vi "Data Analysis.COnvert JSON to CSV.vi"(8 "error in (no error)":errorcluster, 10 "Output Folder":path, 11 "Input Folder":path) -> (0 "error out":errorcluster)   [LabVIEW 2018]
uses:
  Common/Utils/Reports/Report.Result Data JSON V2.0.0.ctl
  Common/Utils/Reports/Report.Result Test Event.ctl
  Common/Utils/Reports/Report.Result State.ctl
  Common/Utils/Reports/Report.Result UUTInfo.ctl
  Common/Utils/Reports/Report.Result Test Station.ctl
  Common/Utils/Reports/Report.Result Test Sequence.ctl
  Common/Utils/Reports/Report.Result Measurement JSON Safe.ctl
  Common/Utils/Reports/Report.Result DataObject.ctl
  <vilib>/KATE/Files/File Utils.lvlib
  <vilib>/zip/NI_Unzip.lvlib
panel:
  in  "Abort":bool
  out "ZipCnt":i32
  out "JSONCnt":i32
  out "ZIP Files In":path[](array[path])
  out "Files Out":path[](array[path])
  out "JSON Files In":path[](array[path])
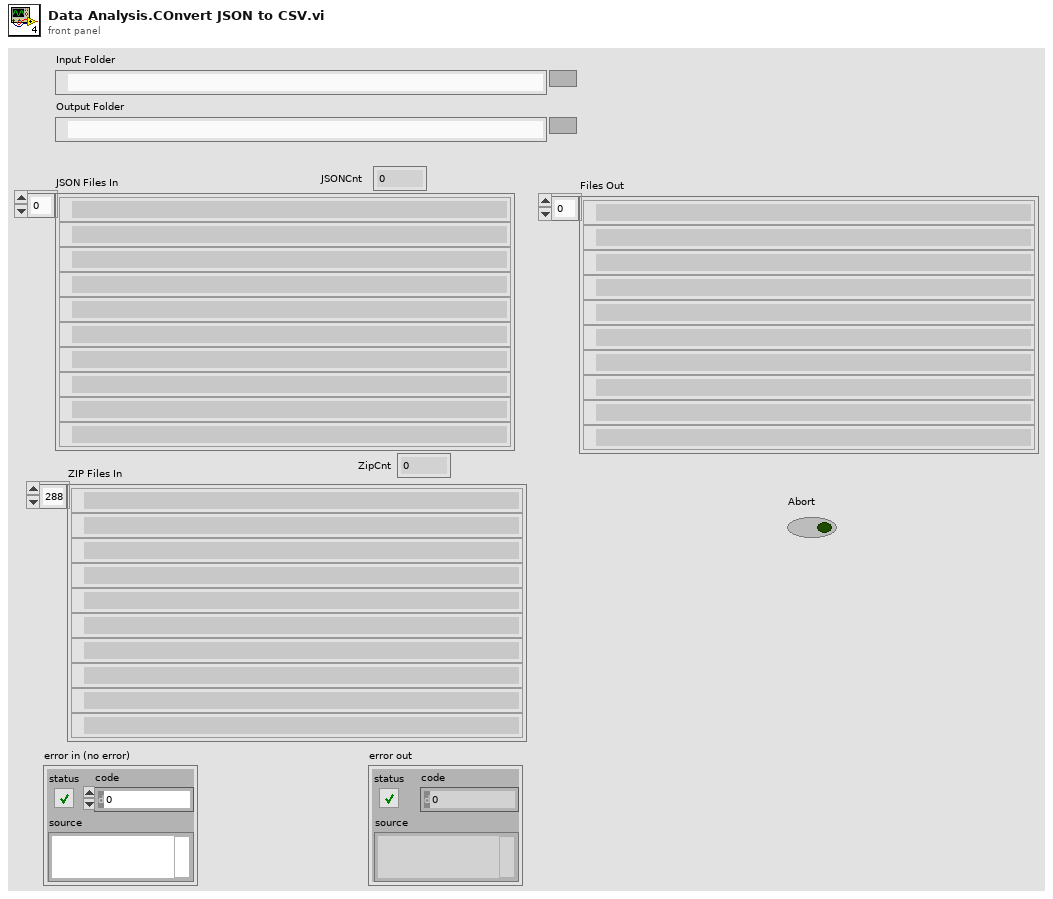
[diagram p1: front panel]
types:
  T1 = typedef "Report.Result Data JSON V2.0.0.ctl" = cluster{"Type":string, "Version":string, "TestEvent":T2, "UUTInfo":T4, "Station":T5, "TestSequence":T6, "ResultData":T7[], "DataObjs":T8[]}
  T2 = typedef "Report.Result Test Event.ctl" = cluster{"ProcessStep":string, "StartTime":string, "EndTime":string, "Mode":string, "Operator":string, "Comment":string, "Result":T3}
  T3 = typedef "Report.Result State.ctl" = cluster{"State":string, "Code":i32, "Desc":string, "Details":string}
  T4 = typedef "Report.Result UUTInfo.ctl" = cluster{"Product":string, "Description":string, "PN":string, "SN":string, "LotNumber":string, "DateCode":string, "AltID":string, "Revision":string, "Properties":cluster{"Name":string, "Value":string}[]}
  T5 = typedef "Report.Result Test Station.ctl" = cluster{"Name":string, "Location":string, "ConfigID":string, "PCName":string, "Slot":string}
  T6 = typedef "Report.Result Test Sequence.ctl" = cluster{"Name":string, "Setup":cluster{"Name":string, "Value":string}[]}
  T7 = typedef "Report.Result Measurement JSON Safe.ctl" = cluster{"Cnt":i32, "Step":string, "Category":string, "Name":string, "Value":string, "Units":string, "LimType":string, "LL":string, "UL":string, "Time":string, "Result":T3}
  T8 = typedef "Report.Result DataObject.ctl" = cluster{"Cnt":i32, "Step":string, "Category":string, "Name":string, "Type":string, "FileName":string, "Time":string}
  T9 = cluster{"JSON Files In":path[], "ZIP Files In":path[]}
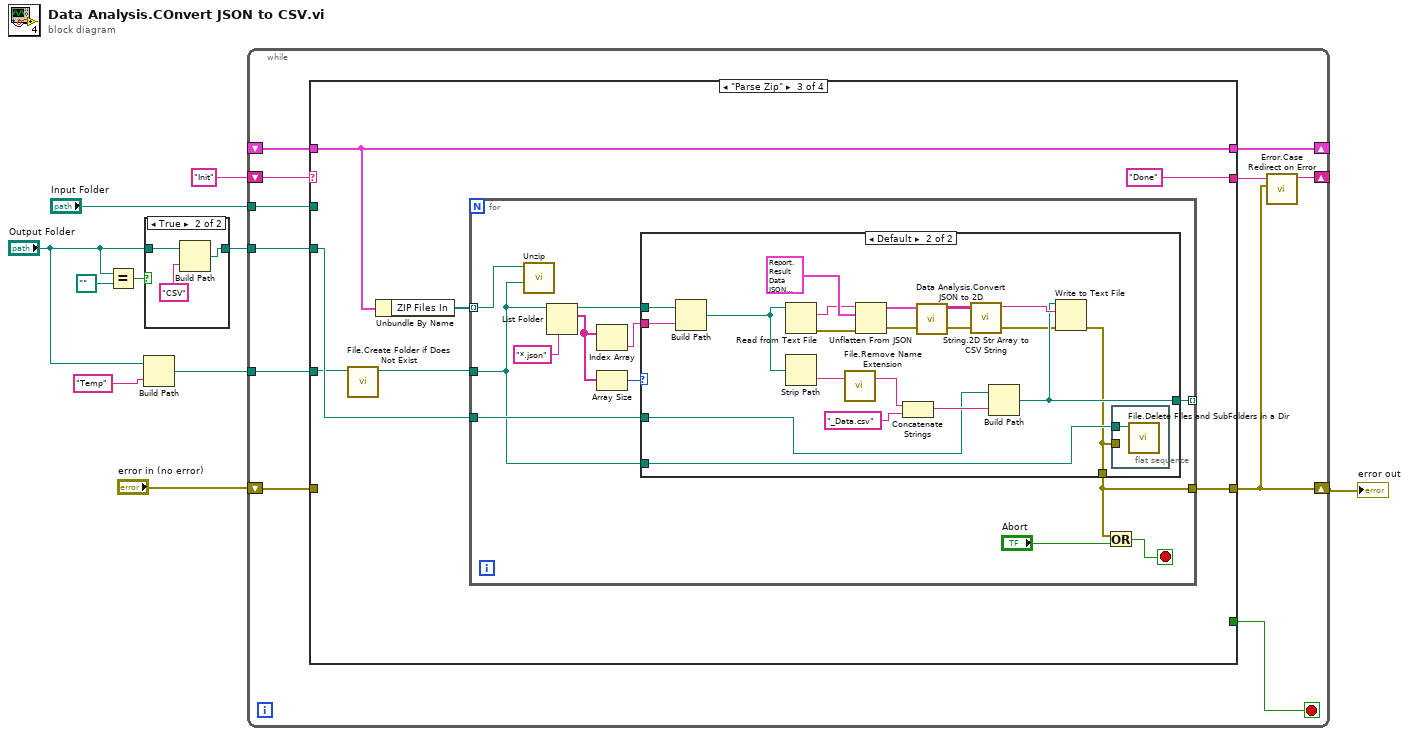
[diagram p0: block diagram]
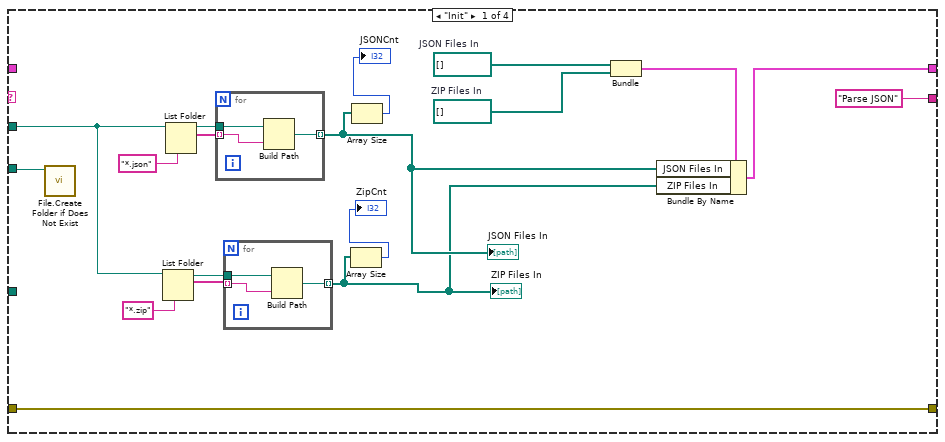
[diagram p3: hidden frame]
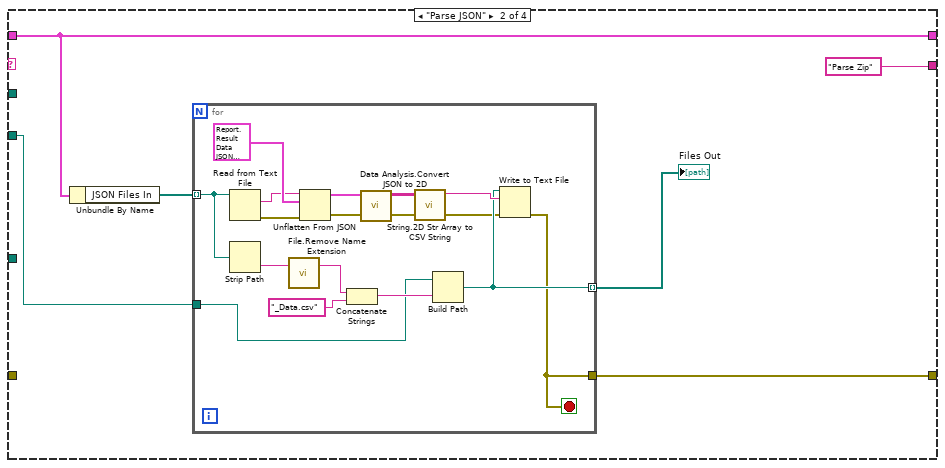
[diagram p4: hidden frame]
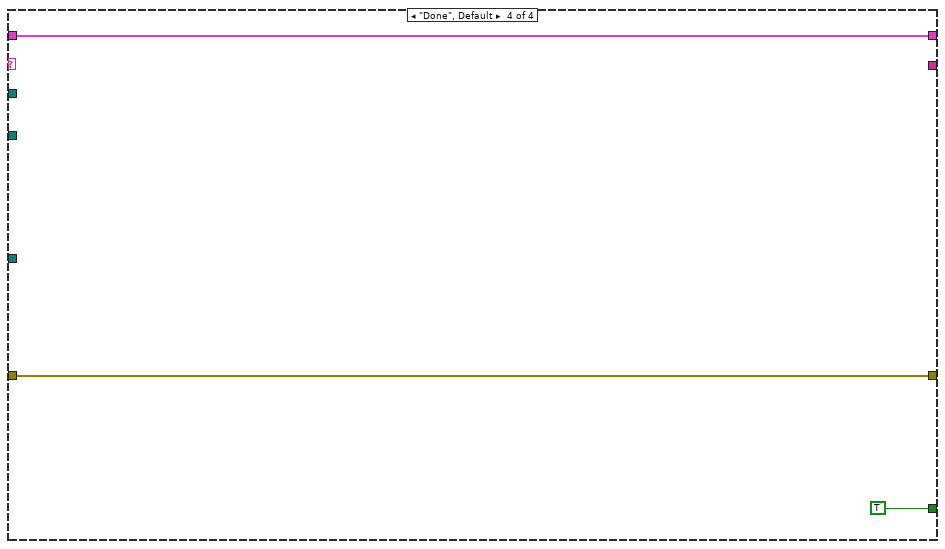
[diagram p6: hidden frame]
diagram:
  n1 = Equal?(x="Output Folder", y=path "") -> (x = y?=w6:bool)
  n2 = Build Path(base path="Output Folder", name or relative path="Temp") -> (appended path=w1:path)
  n3 = case shown="True" w6 {
    tunnel: "Output Folder" -> [w11 w13]
    tunnel: [w11 w12] -> w7
    frame False {
    }
    frame True {
      n4 = Build Path(base path=w13, name or relative path="CSV") -> (appended path=w12:path)
    }
  }
  n5 = while {
    tunnel: "Input Folder" -> [w25]
    tunnel: w7 -> [w24]
    shift-right: [w18] -> _
    shift-left: "Init" -> [w23]
    shift-right: [w21] -> _
    shift-left: _ -> [w20]
    shift-right: [w17] -> w4
    shift-left: "error in (no error)" -> [w16]
    tunnel: w1 -> [w15]
    stop <- w22 stop-if-true
    n6 = case shown="\"Parse Zip\"" w23 {
      tunnel: w25 -> [w40 _ _ _]
      tunnel: w24 -> [w43 w52 w74 _]
      tunnel: ["Parse JSON" "Parse Zip" "Done" _] -> w19
      tunnel: [_ _ _ TRUE] -> w22
      tunnel: [w30 w54 w76 w110] -> w21
      tunnel: w20 -> [_ w54 w76 w110]
      tunnel: [w32 w50 w73 w109] -> w17
      tunnel: w16 -> [w32 _ _ w109]
      tunnel: w15 -> [_ _ w72 _]
      frame "Init" {
        w33 = path[] []  # ZIP Files In
        w34 = path[] []  # JSON Files In
        n7 = call <vilib>:"File.Create Folder if Does Not Exist.vi"("Path"=w43) -> ()  [unwired: 8 in, 3 out]
        n8 = List Folder(path=w40, pattern="*.zip") -> (path out=w37:path, filenames=w36:string[])  [unwired: 2 in, 2 out]
        n9 = List Folder(path=w40, pattern="*.json") -> (path out=w39:path, filenames=w38:string[])  [unwired: 2 in, 2 out]
        n10 = for {
          tunnel: w39 -> [w49]
          tunnel: w38 -> [w48] mode=indexing
          tunnel: [w47] -> w29 mode=indexing
          n11 = Build Path(base path=w49, name or relative path=w48) -> (appended path=w47:path)
        }
        "JSON Files In" <- w29
        n12 = for {
          tunnel: w37 -> [w46]
          tunnel: w36 -> [w45] mode=indexing
          tunnel: [w44] -> w27 mode=indexing
          n13 = Build Path(base path=w46, name or relative path=w45) -> (appended path=w44:path)
        }
        "ZIP Files In" <- w27
        n14 = Array Size(array=w27) -> (size(s)=→"ZipCnt":i32)
        n15 = Array Size(array=w29) -> (size(s)=→"JSONCnt":i32)
        n16 = Bundle("JSON Files In"=w34, "ZIP Files In"=w33) -> (w31:T9)  [unwired: 1 in]
        n17 = Bundle By Name(cluster=w31, "JSON Files In"=w29, "ZIP Files In"=w27) -> (w30:T9)
      }
      frame "Parse JSON" {
        n18 = Unbundle By Name(w54) -> ("JSON Files In"=w53:path[])
        n19 = for {
          tunnel: w53 -> [w66] mode=indexing
          tunnel: w52 -> [w61]
          tunnel: [w58] -> w51 mode=indexing
          tunnel: [w57] -> w50
          stop <- w57 stop-if-true
          n20 = Read from Text File(file (use dialog)=w66) -> (text=w69:string, error out=w68:errorcluster)  [unwired: 3 in, 2 out]
          n21 = Strip Path(path=w66) -> (name=w65:string)  [unwired: 1 out]
          n22 = call <vilib>:"File.Remove Name Extension.vi"("File Name"=w65) -> ("Name Less Ext"=w64:string)  [unwired: 1 in, 1 out]
          n23 = Unflatten From JSON(JSON string=w69, type and defaults=T1 {"Type"="Test Data", "Version"="1.0.0", "TestEvent"={"ProcessStep"="", "StartTime"="", "EndTime"="", "Mode"="", "Operator"="", "Comment"="", "Result"={"State"="", "Code"=0, "Desc"="", "Details"=""}}, "UUTInfo"={"Product"="", "Description"="", "PN"="", "SN"="", "LotNumber"="", "DateCode"="", "AltID"="", "Revision"="", "Properties"=[]}, "Station"={"Name"="", "Location"="", "ConfigID"="", "PCName"="", "Slot"=""}, "TestSequence"={"Name"="", "Setup"=[]}, "ResultData"=[], "DataObjs"=[]} ("Test Result V2"), error in (no error)=w68) -> (value=w67:T1, error out=w56:errorcluster)  [unwired: 4 in]
          n24 = Concatenate Strings(w64, "_Data.csv" ("string")) -> (w62:string)
          n25 = call "Data Analysis.Convert JSON to 2D.vi"("Test Result V2.0.0"=w67) -> ("2D"=w60:string[][])  [unwired: 10 in]
          n26 = call "String.2D Str Array to CSV String.vi"("2D In"=w60) -> ("spreadsheet string"=w59:string)  [unwired: 10 in]
          n27 = Build Path(base path=w61, name or relative path=w62) -> (appended path=w58:path)
          n28 = Write to Text File(file (use dialog)=w58, text=w59, error in=w56) -> (error out=w57:errorcluster)  [unwired: 1 in, 2 out]
        }
        "Files Out" <- w51
      }
      frame "Parse Zip" {
        n29 = call <vilib>:"File.Create Folder if Does Not Exist.vi"("Path"=w72) -> ("Dup Path"=w71:path)  [unwired: 8 in, 2 out]
        n30 = Unbundle By Name(w76) -> ("ZIP Files In"=w75:path[])
        n31 = for {
          tunnel: w75 -> [w87] mode=indexing
          tunnel: w74 -> [w89]
          tunnel: [w88] -> _ mode=indexing
          tunnel: [w80] -> w73
          tunnel: w71 -> [w81]
          stop <- w78 stop-if-true
          n32 = call <vilib>:"Unzip.vi"("Target directory (same as Zip file if empty)"=w81, "Zip file"=w87) -> ()  [unwired: 7 in, 3 out]
          n33 = List Folder(path=w81, pattern="*.json") -> (path out=w84:path, filenames=w83:string[])  [unwired: 2 in, 2 out]
          n34 = Index Array(array=w83) -> (element=w85:string)  [unwired: 1 in]
          n35 = Array Size(array=w83) -> (size(s)=w82:i32)
          n36 = case shown="Default" w82 {
            tunnel: w89 -> [_ w99]
            tunnel: [_ w96] -> w88
            tunnel: [_ w90] -> w80
            tunnel: w85 -> [_ w94]
            tunnel: w84 -> [_ w93]
            tunnel: w81 -> [_ w91]
            frame 0 {
            }
            frame Default {
              n37 = Build Path(base path=w93, name or relative path=w94) -> (appended path=w92:path)
              n38 = Read from Text File(file (use dialog)=w92) -> (text=w106:string, error out=w105:errorcluster)  [unwired: 3 in, 2 out]
              n39 = Strip Path(path=w92) -> (name=w103:string)  [unwired: 1 out]
              n40 = call <vilib>:"File.Remove Name Extension.vi"("File Name"=w103) -> ("Name Less Ext"=w102:string)  [unwired: 1 in, 1 out]
              n41 = Unflatten From JSON(JSON string=w106, type and defaults=T1 {"Type"="Test Data", "Version"="1.0.0", "TestEvent"={"ProcessStep"="", "StartTime"="", "EndTime"="", "Mode"="", "Operator"="", "Comment"="", "Result"={"State"="", "Code"=0, "Desc"="", "Details"=""}}, "UUTInfo"={"Product"="", "Description"="", "PN"="", "SN"="", "LotNumber"="", "DateCode"="", "AltID"="", "Revision"="", "Properties"=[]}, "Station"={"Name"="", "Location"="", "ConfigID"="", "PCName"="", "Slot"=""}, "TestSequence"={"Name"="", "Setup"=[]}, "ResultData"=[], "DataObjs"=[]} ("Test Result V2"), error in (no error)=w105) -> (value=w104:T1, error out=w95:errorcluster)  [unwired: 4 in]
              n42 = Concatenate Strings(w102, "_Data.csv" ("string")) -> (w100:string)
              n43 = call "Data Analysis.Convert JSON to 2D.vi"("Test Result V2.0.0"=w104) -> ("2D"=w98:string[][])  [unwired: 10 in]
              n44 = call "String.2D Str Array to CSV String.vi"("2D In"=w98) -> ("spreadsheet string"=w97:string)  [unwired: 10 in]
              n45 = Build Path(base path=w99, name or relative path=w100) -> (appended path=w96:path)
              n46 = Write to Text File(file (use dialog)=w96, text=w97, error in=w95) -> (error out=w90:errorcluster)  [unwired: 1 in, 2 out]
              n47 = flat-sequence {
                tunnel: w91 -> [w108]
                tunnel: w90 -> [_]
                frame #0 {
                  n48 = call <vilib>:"File.Delete Files and SubFolders in a Dir.vi"("Dir"=w108) -> ()  [unwired: 9 in, 2 out]
                }
              }
            }
          }
          n49 = Or(x=w80, y="Abort") -> (x .or. y?=w78:bool)
        }
      }
      frame "Done", Default {
      }
    }
    n50 = call "Error.Case Redirect on Error.vi"("error in"=w17, "Next Case"=w19) -> ("Next Case Out"=w18:string)  [unwired: 9 in]
  }
  "error out" <- w4
